vi "Update activity log cluster array.vi"(4 "Activity description":string, 5 "Activity log in":T1 {"Epoch sec" format="%.2e"}) -> (2 "Activity log out":T1 {"Epoch sec" format="%.2e"})   [LabVIEW 2013]
doc: "Adds an element to the end of the input activity cluster array. Uses the current epoch seconds from the PC clock and the input \"activity description\" to create the new element."
uses:
  User Access Type defs/Acitivity cluster array.ctl
  User Access Type defs/Acitivity cluster.ctl
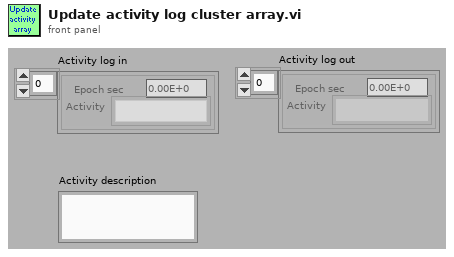
[diagram p1: front panel]
types:
  T1 = typedef "Acitivity cluster array.ctl" = T2[]
  T2 = typedef "Acitivity cluster.ctl" = cluster{"Epoch sec":dbl, "Activity":string}
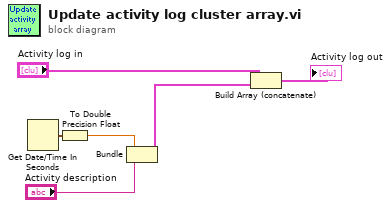
[diagram p0: block diagram]
diagram:
  n1 = Get Date/Time In Seconds() -> (seconds since 1Jan1904=w1:timestamp)
  n2 = To Double Precision Float(number=w1) -> (double precision float=w5:dbl)
  n3 = Bundle(w5, "Activity description"="Activity description") -> (w3:cluster{dbl, "Activity description":string})  [unwired: 1 out]
  n4 = Build Array (concatenate)("Activity log in", w3) -> (→"Activity log out":T1)
